vi "FPGA cRIOMain_v11.vi"() -> ()   [LabVIEW 2019]
doc: "Main FPGA VI\nUse the bitfile generated by this VI in the real-time code.\n\nv5: Use 16-pt MA filter in AI loop"
uses:
  TypeDefs/AO mode TabCtrl.ctl
  TypeDefs/AI_channelEnum.ctl
  TypeDefs/SamplingModeEnum_v2.ctl
  <vilib>/Platform/TimedLoop/XDataNode/timing_clust.ctl
  <vilib>/Platform/TimedLoop/XDataNode/nitl_modes.ctl
  <vilib>/Platform/TimedLoop/XDataNode/wakeup.ctl
  <vilib>/rvi/Emulation/niFpgaGetClockAttributes.vi
  <vilib>/rvi/Emulation/niFpgaSctlEmulationGetInTimedLoop.vi
  <vilib>/rvi/Emulation/niFpgaEmulationReportErrorSimple.vi
  <vilib>/rvi/eio/common/nirviEmuTemplateMethod_errors.vi
  <vilib>/rvi/Emulation/niFpgaEmulationIsFPGAContextNoSignature.vi
  <vilib>/rvi/errors/niFpgaSetErrorForExecOnDevCompSimple.vi
  <vilib>/rvi/eio/common/nirviEmuReportErrorAndStop.vi
  <vilib>/rvi/DataTransferAndStorage/Container/Common/niFpgaContainerGetUniqueNameForEmu.vi
  <vilib>/rvi/FIFO/Fifo_Resource/nirvififoEmulationSetSize.vi
  <vilib>/rvi/FIFO/Fifo_Resource/nirviFifoEmulationQueueMgr.vi
  <instcachedir>/0/nirviFifoEmulationQueueMgr_E5CAEC123FF24DC58D834DCA3CDAA9B5.lvgen/nirviFifoEmulationQueueMgr_E5CAEC123FF24DC58D834DCA3CDAA9B5_000.vi
  <vilib>/rvi/FIFO/Fifo_Resource/nirvififoEmulationDetermineInputValidOut.vi
  <vilib>/rvi/FIFO/Fifo_Resource/nirvififoEmulationCreateLock.vi
  <vilib>/rvi/Emulation/niFpgaProcessEmulError.vi
  <vilib>/rvi/FIFO/Fifo_Resource/nirvififoEmulationObtainLock.vi
  <vilib>/rvi/FIFO/Fifo_Resource/nirvififoEmulationReleaseLock.vi
  <vilib>/rvi/occurrence/nirviWaitOnOccurrenceBase.vi
  <vilib>/rvi/errors/nirviReportUnexpectedCaseInternalError.vi
  <vilib>/rvi/errors/nirviReportUnexpectedCaseInternalError (U32).vi
  <vilib>/rvi/Emulation/niFpgaCriticalErrorInLSC.vi
  <instcachedir>/0/nirviFifoEmulationQueueMgr_E5CAEC123FF24DC58D834DCA3CDAA9B5.lvgen/nirviFifoEmulationQueueMgr_E5CAEC123FF24DC58D834DCA3CDAA9B5_006.vi
  <vilib>/Utility/error.llb/Clear Errors.vi
  <vilib>/rvi/Analysis/common/codeGenErrors/XNode/niFpgaXNodeCodeGenErrorHandle.vi
  <vilib>/eio/EIONode/EIONode.xnode
  <vilib>/rvi/DataTransferAndStorage/Container/XNode/niFpgaContainer.xnode
  <vilib>/rvi/FIFO/Fifo_Resource/nirvififoEmulationWrite.vi
  <vilib>/rvi/FIFO/Fifo_Resource/nirvififoEmulationRead.vi
  <vilib>/rvi/Analysis/measure/butterworth/XNode/niFpgaButterworthFilter.xnode
  <vilib>/rvi/FXPMathLib/FxpMul/XNode/nifxpmath_Multiplier.xnode
  <vilib>/rvi/Analysis/measure/LMRsmpl/XNode/niFPGA Rational Resampler.xnode
  <vilib>/Platform/TimedLoop/XDataNode/XDataNode.xnode
  FPGA functions/FPGA functions.lvlib
  <vilib>/Platform/TimedLoop/XDataNode/XDNodeRunTimeDep.lvlib
  <vilib>/rvi/FXPMathLib/sim/FxpSim.dll
panel:
  in  "scaled BW coefficients":i32[](array[numeric])=[-850883994, 1909449570, 3794062, -975456236, 2033039520, 4039635]
  in  "Sampling Mode":T1
  out "AI M loop time [ticks]":u32
  out "FPGA AI DMA\nOverflow?":bool
  out "AI Processing\nLoop Rate to high?":bool
  in  "AI Process Time [ticks]":u32=125
  in  "Select Channel":T2
  out "Unable to\nsample at desired\nSample Rate?":bool
  out "Processing Loop time [ticks]":u32
  in  "AO mode":T3
  in  "AO Out [V]":fxp<+/-,18,5> format="%#.6g"
  in  "AO enable?":bool
  out "AI In [V]":fxp<+/-,28,5> format="%#.6g"
  out "FPGA AO DMA\nOverflow?":bool
  out "Int. Output":fxp<+/-,20,5> format="%.17g"
  out "Raw AI Input":fxp<+/-,28,5> format="%.21g"
  in  "Sample Time [ticks]":u32=125
  out "AO Loop time [ticks]":u32
  out "AI Loop time [ticks]":u32
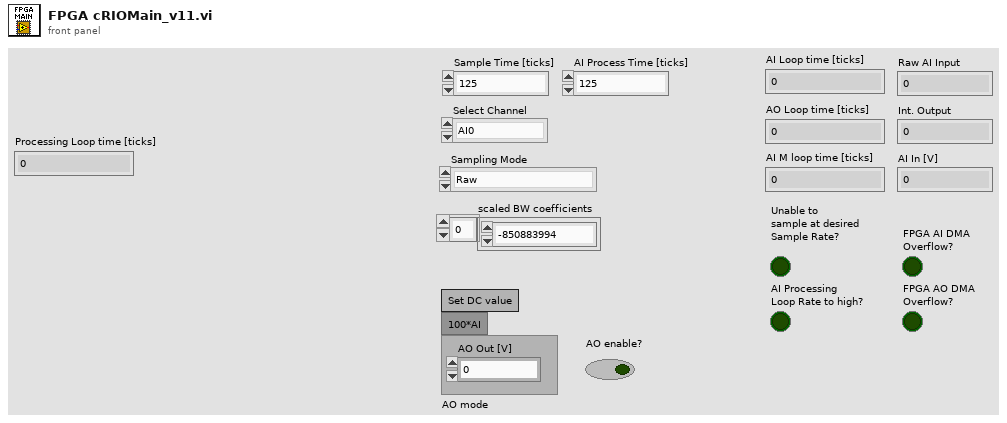
[diagram p1: front panel]
types:
  T1 = typedef "SamplingModeEnum_v2.ctl" = enum16{"Raw", "M64 - Resampling", "2nd-order Butterworth", "4th-order Butterworth", "64pt-MA", "128pt-MA", "256pt-MA"}
  T2 = typedef "AI_channelEnum.ctl" = enum16{"AI0", "AI1", "AI2", "AI3"}
  T3 = typedef "AO mode TabCtrl.ctl" = enum32{"Set DC value", "100*AI"}
  T4 = typedef "XDNodeRunTimeDep.lvlib/timing_clust.ctl" = cluster{"Expected End [f-1]":u64, "Actual End [f-1]":u64, "Finished Late? [f-1]":bool, "Expected End [i-1]":u64, "Actual End [i-1]":u64, "Finished Late? [i-1]":bool, "Expected Start [i]":u64, "Actual Start [i]":u64, "Expected Start [f]":u64, "Actual Start [f]":u64, "Source Name":string, "Structure Name":string, "Period":i64, "Deadline":i64, "Offset":i64, "Start":i64, "Priority":i32, "Timeout":i32, "Mode":T5, "Wakeup Reason":T6, "Error":errorcluster, "Source Type":string, "Secondary Source Type":string, "Global End Time":u64, "Global Start Time":u64, "Frame Duration":u64, "Iteration Duration":u64, "Assigned CPU":i32, "I/O Scan Engine Mode":u32}
  T5 = typedef "XDNodeRunTimeDep.lvlib/nitl_modes.ctl" = enum32{"No Change", "Process missed periods, maintain original phase", "Discard missed periods, maintain original phase", "Process missed periods, ignore original phase", "Discard missed periods, ignore original phase"}
  T6 = typedef "XDNodeRunTimeDep.lvlib/wakeup.ctl" = enum32{"Normal", "Aborted", "Asynchronous wakeup", "Timing source error", "Timed loop error", "Timeout"}
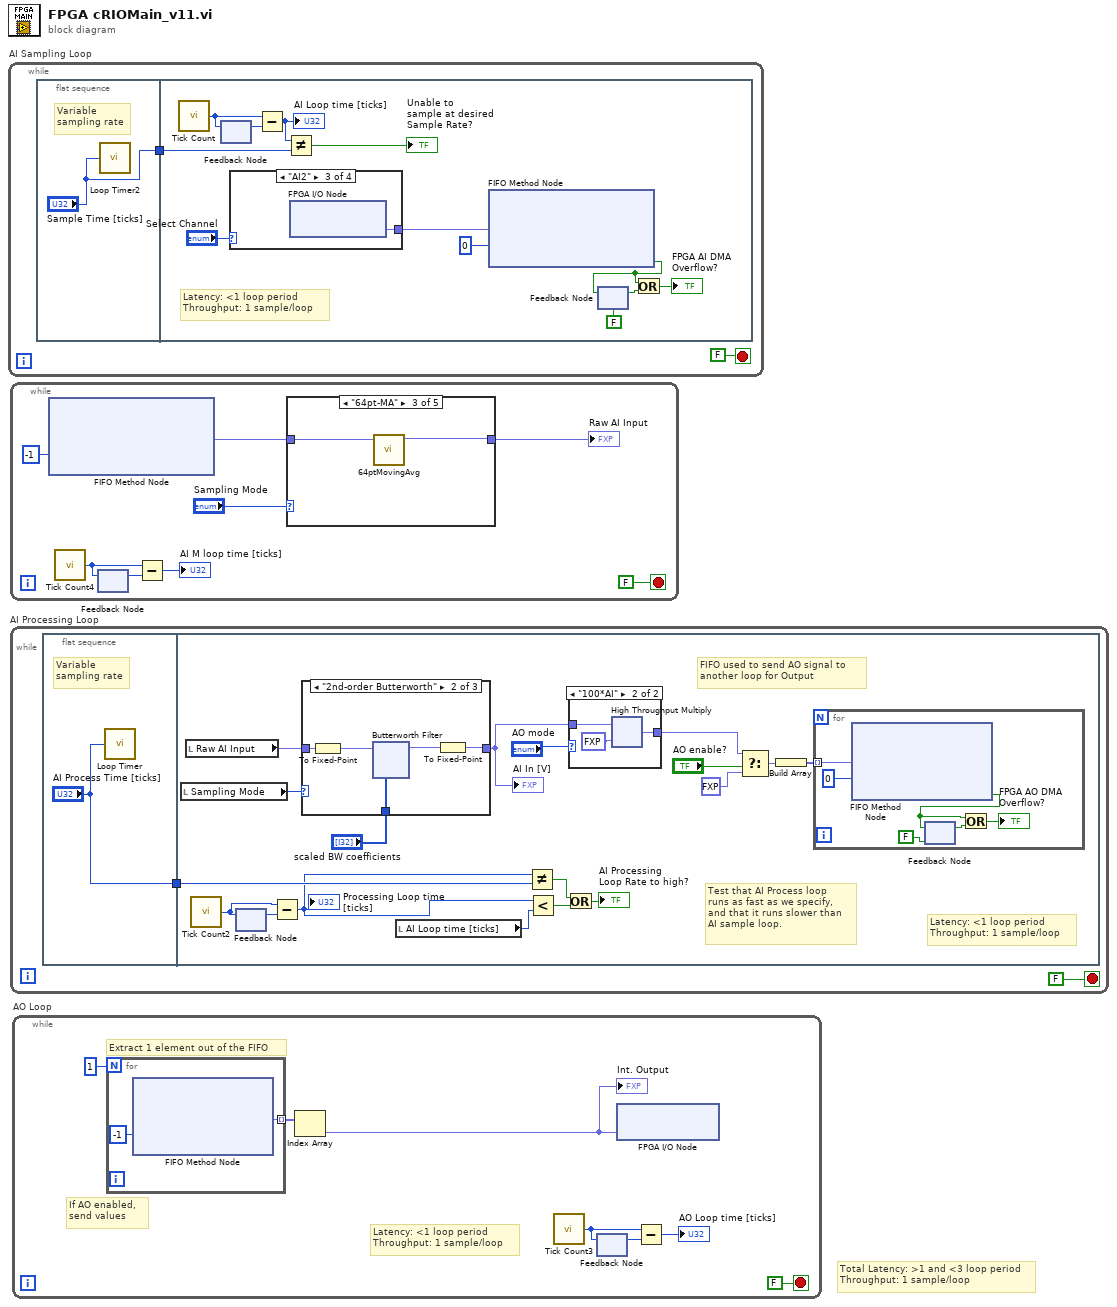
[diagram p0: block diagram]
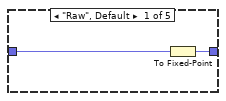
[diagram p2: hidden frame]
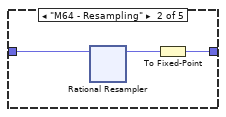
[diagram p3: hidden frame]
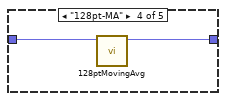
[diagram p4: hidden frame]
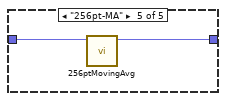
[diagram p5: hidden frame]
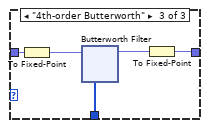
[diagram p7: hidden frame]
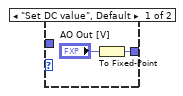
[diagram p8: hidden frame]
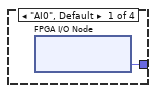
[diagram p9: hidden frame]
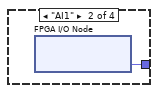
[diagram p10: hidden frame]
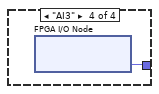
[diagram p11: hidden frame]
diagram:
  # "Total Latency: >1 and <3 loop period\nThroughput: 1 sample/loop"
  n1 = while "AI Sampling Loop" {
    stop <- FALSE stop-if-true
    n2 = flat-sequence {
      tunnel: ["Sample Time [ticks]"] -> w1
      tunnel: w1 -> [w12]
      frame #0 {
        # "Variable\nsampling rate"
        n3 = call "Loop Timer2"("Count(Ticks)"="Sample Time [ticks]") -> ()  [unwired: 1 out]
      }
      frame #1 {
        # "Latency: <1 loop period\nThroughput: 1 sample/loop"
        n4 = call "Tick Count"() -> ("Tick Count(Ticks)"=w15:u32)
        n5 = feedback #1() -> (w14:u32)  [unwired: 1 in]
        n6 = feedback-in #1(w15) -> ()
        n7 = case shown="\"AI2\"" "Select Channel" {
          tunnel: [w16 w17 w18 w19] -> w4
          frame "AI0", Default {
            n8 = xnode "FPGA I/O Node"() -> ("Mod4/AI0"=w16:fxp<+/-,24,5>)  [unwired: 1 in, 1 out]
          }
          frame "AI1" {
            n9 = xnode "FPGA I/O Node"() -> ("Mod4/AI1"=w17:fxp<+/-,24,5>)  [unwired: 1 in, 1 out]
          }
          frame "AI2" {
            n10 = xnode "FPGA I/O Node"() -> ("Mod4/AI2"=w18:fxp<+/-,24,5>)  [unwired: 1 in, 1 out]
          }
          frame "AI3" {
            n11 = xnode "FPGA I/O Node"() -> ("Mod4/AI3"=w19:fxp<+/-,24,5>)  [unwired: 1 in, 1 out]
          }
        }
        n12 = Subtract(x=w15, y=w14) -> (x-y=w13:u32)
        "AI Loop time [ticks]" <- w13
        n13 = Not Equal?(x=w13, y=w12) -> (x != y?=→"Unable to\nsample at desired\nSample Rate?":bool)
        n14 = xnode ("FIFO Method Node")("Element"=w4, "Timeout"=0) -> ("Timed Out?"=w7:bool)  [unwired: 1 in, 1 out]
        n15 = feedback #2(FALSE ("Timed Out?")) -> (w9:bool)
        n16 = feedback-in #2(w7) -> ()
        n17 = Or(x=w7, y=w9) -> (x .or. y?=→"FPGA AI DMA\nOverflow?":bool)
      }
    }
  }
  n18 = while {
    stop <- FALSE stop-if-true
    n19 = xnode ("FIFO Method Node")("Timeout"=-1) -> ("Element"=w21:fxp<+/-,24,5>)  [unwired: 1 in, 2 out]
    n20 = call "Tick Count4"() -> ("Tick Count(Ticks)"=w25:u32)
    n21 = feedback #3() -> (w24:u32)  [unwired: 1 in]
    n22 = feedback-in #3(w25) -> ()
    n23 = Subtract(x=w25, y=w24) -> (x-y=→"AI M loop time [ticks]":u32)
    n24 = case shown="\"64pt-MA\"" "Sampling Mode" {
      tunnel: w21 -> [w28 w32 w68 w70 w71]
      tunnel: [w29 w31 w67 w69 w72] -> w20
      frame "Raw", Default {
        n25 = To Fixed-Point(number=w28) -> (fixed-point=w29:fxp<+/-,28,5>)  [unwired: 1 in]
      }
      frame "M64 - Resampling" {
        n26 = xnode "Rational Resampler"("input data"=w32) -> ("output data"=w30:fxp<+/-,26,5>)  [unwired: 2 out]
        n27 = To Fixed-Point(number=w30) -> (fixed-point=w31:fxp<+/-,28,5>)  [unwired: 1 in]
      }
      frame "64pt-MA" {
        n28 = call "64ptMovingAvg.vi"("Raw input"=w68) -> ("Output"=w67:fxp<+/-,28,5>)  [unwired: 10 in]
      }
      frame "128pt-MA" {
        n29 = call "128ptMovingAvg.vi"("Raw input"=w70) -> ("Output"=w69:fxp<+/-,28,5>)  [unwired: 10 in]
      }
      frame "256pt-MA" {
        n30 = call "256ptMovingAvg.vi"("Raw input"=w71) -> ("Output"=w72:fxp<+/-,28,5>)  [unwired: 10 in]
      }
    }
    "Raw AI Input" <- w20
  }
  n31 = while "AI Processing Loop" {
    stop <- FALSE stop-if-true
    n32 = flat-sequence {
      tunnel: ["AI Process Time [ticks]"] -> w73
      tunnel: w73 -> [w81]
      frame #0 {
        # "Variable\nsampling rate"
        n33 = call "Loop Timer"("Count(Ticks)"="AI Process Time [ticks]") -> ()  [unwired: 1 out]
      }
      frame #1 {
        # "Test that AI Process loop\nruns as fast as we specify,\nand that it runs slower than \nAI sample loop."
        # "Latency: <1 loop period\nThroughput: 1 sample/loop"
        # "FIFO used to send AO signal to \nanother loop for Output"
        n34 = local read "Sampling Mode"() -> (w79:T1)
        n35 = local read "Raw AI Input"() -> (w78:fxp<+/-,28,5>)
        n36 = call "Tick Count2"() -> ("Tick Count(Ticks)"=w92:u32)
        n37 = feedback #4() -> (w93:u32)  [unwired: 1 in]
        n38 = feedback-in #4(w92) -> ()
        n39 = Subtract(x=w92, y=w93) -> (x-y=w80:u32)
        "Processing Loop time [ticks]" <- w80
        n40 = case shown="\"2nd-order Butterworth\"" w79 {
          tunnel: w78 -> [w94 w97 w110]
          tunnel: [w94 w98 w111] -> w77
          tunnel: "scaled BW coefficients" -> [_ w95 w108]
          frame "Raw", Default {
          }
          frame "2nd-order Butterworth" {
            n41 = To Fixed-Point(number=w97) -> (fixed-point=w96:fxp<+/-,24,5>)  [unwired: 1 in]
            n42 = xnode "Butterworth Filter"("input data"=w96, "scaled coefficients"=w95) -> ("output data"=w99:fxp<+/-,28,9>)  [unwired: 1 in]
            n43 = To Fixed-Point(number=w99) -> (fixed-point=w98:fxp<+/-,28,5>)  [unwired: 1 in]
          }
          frame "4th-order Butterworth" {
            n44 = To Fixed-Point(number=w110) -> (fixed-point=w109:fxp<+/-,24,5>)  [unwired: 1 in]
            n45 = xnode "Butterworth Filter"("input data"=w109, "scaled coefficients"=w108) -> ("output data"=w112:fxp<+/-,28,9>)  [unwired: 1 in]
            n46 = To Fixed-Point(number=w112) -> (fixed-point=w111:fxp<+/-,28,5>)  [unwired: 1 in]
          }
        }
        "AI In [V]" <- w77
        n47 = local read "AI Loop time [ticks]"() -> (w85:u32)
        n48 = Not Equal?(x=w80, y=w81) -> (x != y?=w83:bool)
        n49 = Less?(x=w80, y=w85) -> (x < y?=w82:bool)
        n50 = Or(x=w83, y=w82) -> (x .or. y?=→"AI Processing\nLoop Rate to high?":bool)
        n51 = case shown="\"100*AI\"" "AO mode" {
          tunnel: [w122 w124] -> w89
          tunnel: w77 -> [_ w123]
          frame "Set DC value", Default {
            n52 = To Fixed-Point(number="AO Out [V]") -> (fixed-point=w122:fxp<+/-,20,5>)  [unwired: 1 in]
          }
          frame "100*AI" {
            n53 = xnode ("High Throughput Multiply")("x"=w123, "y"=fxp<+,5,7> 100.0) -> ("x*y"=w124:fxp<+/-,20,5>)
          }
        }
        n54 = Select(t=w89, s="AO enable?", f=fxp<+/-,20,5> 0.0) -> (s? t:f=w91:fxp<+/-,20,5>)
        n55 = Build Array(w91) -> (w88:fxp<+/-,20,5>[])
        n56 = for {
          tunnel: w88 -> [w126] mode=indexing
          n57 = xnode ("FIFO Method Node")("Element"=w126, "Timeout"=0) -> ("Timed Out?"=w127:bool)  [unwired: 1 in, 1 out]
          n58 = feedback-in #5(w127) -> ()
          n59 = feedback #5(FALSE ("Timed Out?")) -> (w130:bool)
          n60 = Or(x=w127, y=w130) -> (x .or. y?=→"FPGA AO DMA\nOverflow?":bool)
        }
      }
    }
  }
  n61 = while "AO Loop" {
    stop <- FALSE stop-if-true
    # "Latency: <1 loop period\nThroughput: 1 sample/loop"
    # "If AO enabled, \nsend values"
    # "Extract 1 element out of the FIFO"
    n62 = for {
      N: 1 -> [_]
      tunnel: [w140] -> w134 mode=indexing
      n63 = xnode ("FIFO Method Node")("Timeout"=-1) -> ("Element"=w140:fxp<+/-,20,5>)  [unwired: 1 in, 2 out]
    }
    n64 = Index Array(array=w134) -> (element=w132:fxp<+/-,20,5>)  [unwired: 1 in]
    "Int. Output" <- w132
    n65 = call "Tick Count3"() -> ("Tick Count(Ticks)"=w137:u32)
    n66 = feedback #6() -> (w136:u32)  [unwired: 1 in]
    n67 = feedback-in #6(w137) -> ()
    n68 = xnode "FPGA I/O Node"("Mod3/AO1"=w132) -> ()  [unwired: 1 in, 1 out]
    n69 = Subtract(x=w137, y=w136) -> (x-y=→"AO Loop time [ticks]":u32)
  }
